vi "path__v1.vi"(0 "光線ベクトル[n-1]":ext[][](array[numeric]), 1 "D":ext, 2 "R":ext, 3 "n":ext) -> (4 "光線ベクトル[n]":ext[][](array[numeric]))   [LabVIEW 2020]
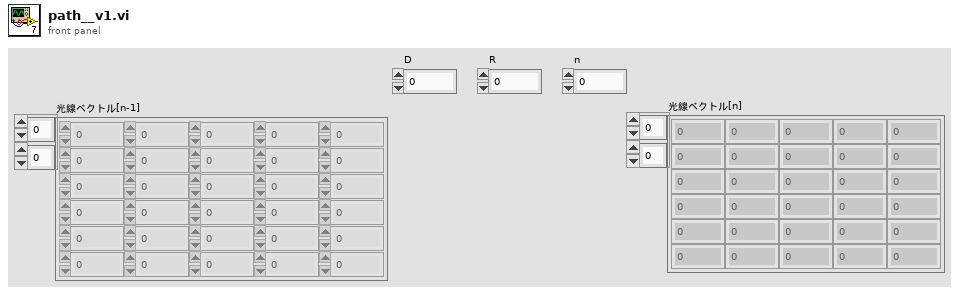
[diagram p1: front panel]
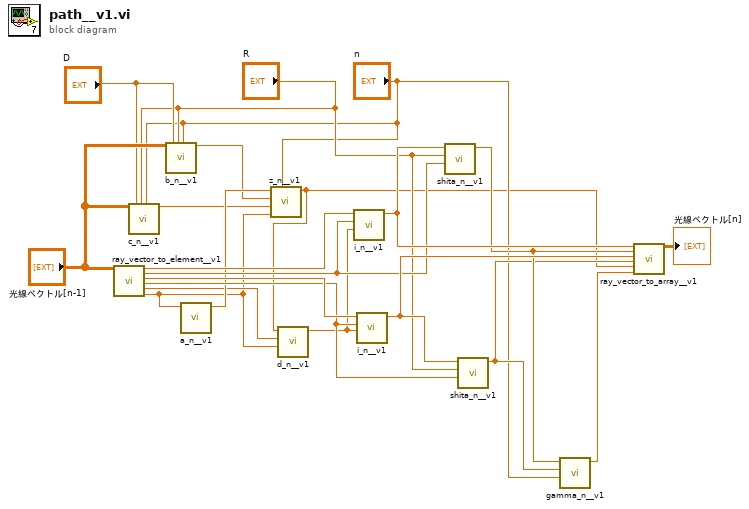
[diagram p0: block diagram]
diagram:
  n1 = call "ray_vector_to_element__v1.vi"("光線ベクトル"="光線ベクトル[n-1]") -> ("x"=w21:ext, "α"=w13:ext, "y"=w20:ext, "β"=w12:ext, "z"=w4:ext, "γ"=w3:ext)  [unwired: 13 in]
  n2 = call "c_n__v1.vi"("配列"="光線ベクトル[n-1]", "D"="D", "R"="R", "n"="n") -> ("c[n]"=w6:ext)  [unwired: 15 in]
  n3 = call "b_n__v1.vi"("光線ベクトル[n-1]"="光線ベクトル[n-1]", "D"="D", "R"="R", "n"="n") -> ("b[n]"=w7:ext)  [unwired: 15 in]
  n4 = call "a_n__v1.vi"("γ[n-1]"=w3) -> ("a[n]"=w8:ext)  [unwired: 10 in]
  n5 = call "z_n__v1.vi"("n"="n", "γ[n-1]"=w3, "c[n]"=w6, "b[n]"=w7, "a[n]"=w8) -> ("z[n]"=w2:ext)  [unwired: 6 in]
  n6 = call "d_n__v1.vi"("γ[n-1]"=w3, "z[n-1]"=w4, "z[n]"=w2) -> ("d[n]"=w1:ext)  [unwired: 8 in]
  n7 = call "i_n__v1.vi"("d[n]"=w1, "θ[n-1]"=w13, "i[n-1]"=w21) -> ("i[n]"=w18:ext)  [unwired: 8 in]
  n8 = call "i_n__v1.vi"("d[n]"=w1, "θ[n-1]"=w12, "i[n-1]"=w20) -> ("i[n]"=w17:ext)  [unwired: 8 in]
  n9 = call "shita_n__v1.vi"("θ[n-1]"=w13, "R"="R", "i[n]"=w18) -> ("θ[n]"=w16:ext)  [unwired: 8 in]
  n10 = call "shita_n__v1.vi"("θ[n-1]"=w12, "R"="R", "i[n]"=w17) -> ("θ[n]"=w15:ext)  [unwired: 8 in]
  n11 = call "gamma_n__v1.vi"("n"="n", "β[n]"=w15, "α[n]"=w16) -> ("γ[n]"=w14:ext)  [unwired: 8 in]
  n12 = call "ray_vector_to_array__v1.vi"("x"=w18, "α"=w16, "y"=w17, "β"=w15, "z"=w2, "γ"=w14) -> ("光線ベクトル"=→"光線ベクトル[n]":ext[][])  [unwired: 13 in]
